vi "TranslateScanCodes.vi"(11 "ScanCode in":i16) -> (3 "ScanCode out":i16)   [LabVIEW 2022 SP3]
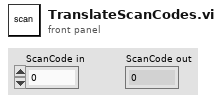
[diagram p1: front panel]
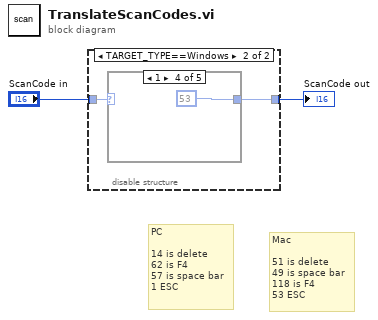
[diagram p0: block diagram]
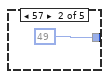
[diagram p4: hidden frame]
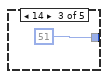
[diagram p5: hidden frame]
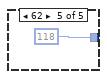
[diagram p6: hidden frame]
diagram:
  # "Mac\n\n51 is delete\n49 is space bar\n118 is F4\n53 ESC"
  # "PC\n\n14 is delete\n62 is F4\n57 is space bar\n1 ESC"
  n1 = disable-structure shown="TARGET_TYPE==Windows" {
    disable-tunnel: [w3 w4] -> w1
    disable-tunnel: "ScanCode in" -> [w3 w5]
    frame condition #0 (active) {
    }
    frame condition #1 {
      n2 = case shown="1" w5 {
        selector: w5 -> [w6 _ _ _ _]
        tunnel: [w6 49 51 53 118] -> w4
        frame 0, Default {
        }
        frame 57 {
        }
        frame 14 {
        }
        frame 1 {
        }
        frame 62 {
        }
      }
    }
  }
  "ScanCode out" <- w1
